vi "WaveGraph_Facade.vi"(0 "Data In":T5 caption="数据输入", 2 "Display State In":T3 caption="显示状态输入", 3 "Container State":T4 caption="容器状态") -> (6 "Data Out":T5 caption="数据输出", 7 "Display State Out":T3 caption="显示状态输出", 8 "Action":T2 caption="动作")   [LabVIEW 2012, in "WaveGraphX.xctl"]
uses:
  WaveGraphX.xctl
  WaveGrpah_Data.ctl
  <vilib>/_xctls/Container State.ctl
  WaveGraph_State.ctl
  <vilib>/Utility/miscctls.llb/LVPoint32TypeDef.ctl
  <vilib>/_xctls/Action.ctl
  <vilib>/_xctls/XControlSupport.lvlib
panel:
  out "峰值图例拖动State":bool
  out "统计图例拖动State":bool
  out "峰值图例":picture
  out "统计图例":picture
  out "图例拖动State":bool
  out "图例":picture
  out "队列中元素数量":i32
  in  "图例拖动坐标队列":refnum<queue>
  out "坐标 2":T1 caption="坐标"
  out "项标识符":string
  out "WaveForm Graph":dbl[](graph)
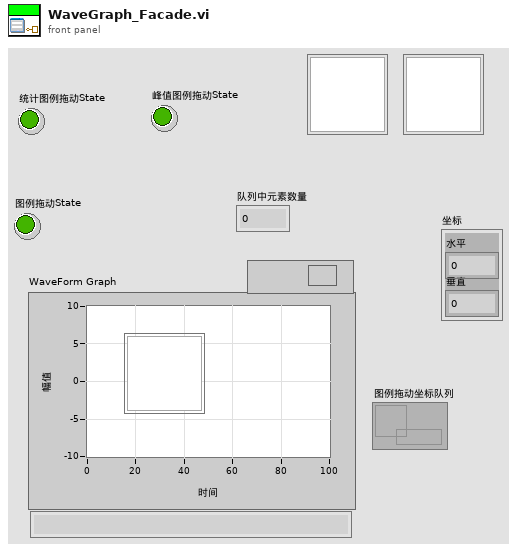
[diagram p1: front panel]
types:
  T1 = typedef "LVPoint32TypeDef.ctl" = cluster{"Horizontal":i32, "Vertical":i32}
  T2 = typedef "XControlSupport.lvlib/Action.ctl" = cluster{"Data Changed?":bool, "State Changed?":bool, "Action Name":string}
  T3 = typedef "WaveGraphX.xctl/WaveGraph_State.ctl" = cluster{"图例拖动State":bool, "统计图例拖动State":bool, "峰值图例拖动State":bool, "图例拖动坐标 队列":refnum<queue>, "统计图例拖动坐标 队列":refnum<queue>, "峰值图例拖动坐标 队列":refnum<queue>, "后台服务VI 引用":refnum<vi>, "控件引用簇 队列":refnum<queue>}
  T4 = typedef "XControlSupport.lvlib/Container State.ctl" = cluster{"Indicator?":bool, "Run Mode?":bool, " Refnum":refnum<vi>}
  T5 = typedef "WaveGraphX.xctl/WaveGrpah_Data.ctl" = dbl[]
  T6 = cluster{"图例拖动State":refnum<vi>, "统计图例拖动State":refnum<vi>, "峰值图例拖动State":refnum<vi>, "图例":refnum<vi>, "统计图例":refnum<vi>, "峰值图例":refnum<vi>}
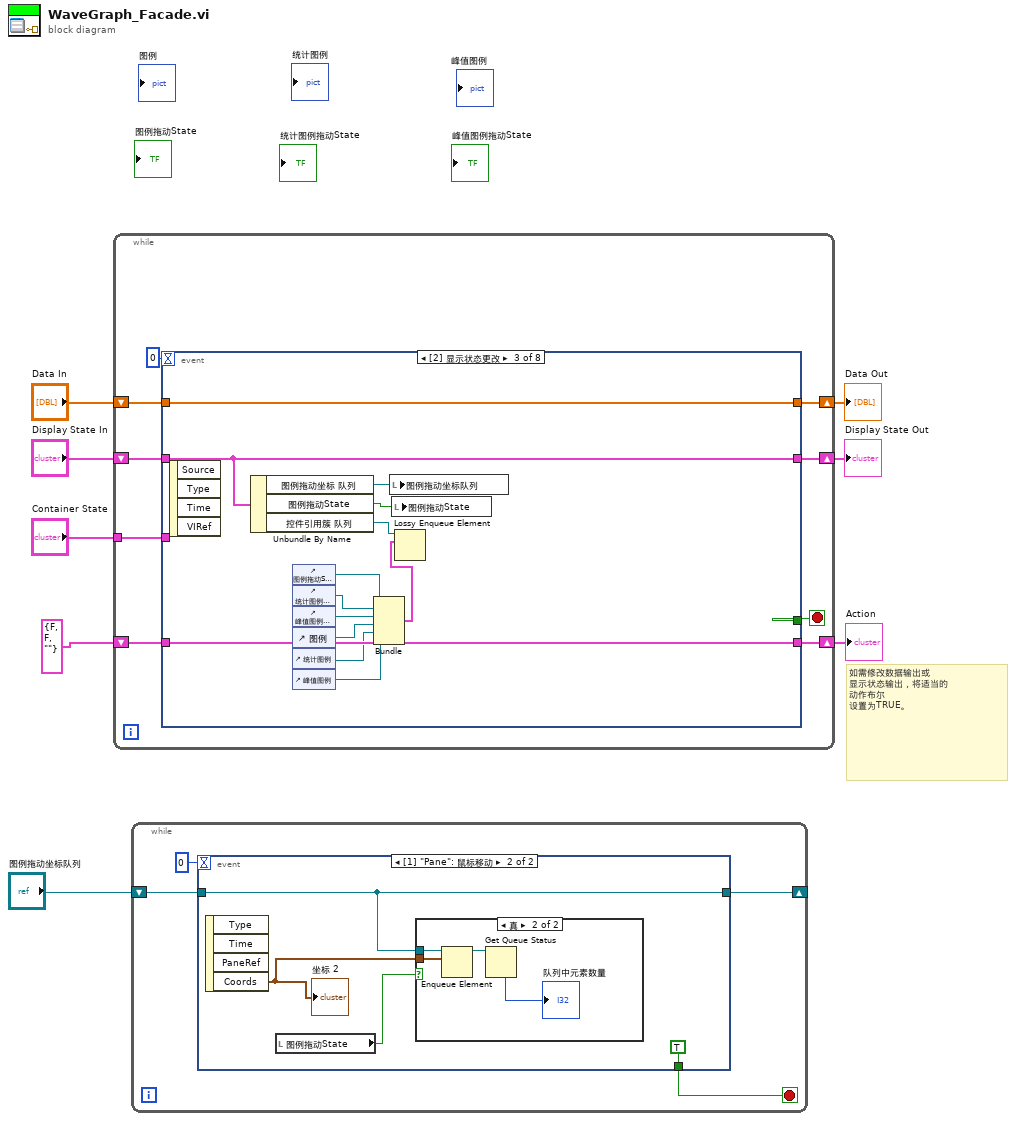
[diagram p0: block diagram]
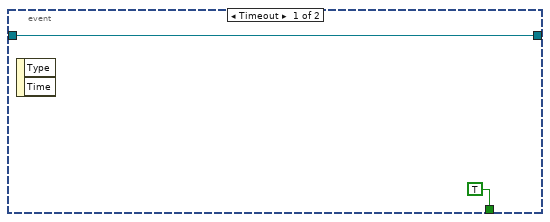
[diagram p2: hidden frame]
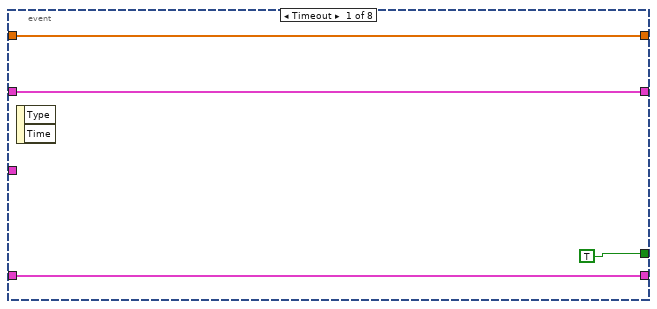
[diagram p4: hidden frame]
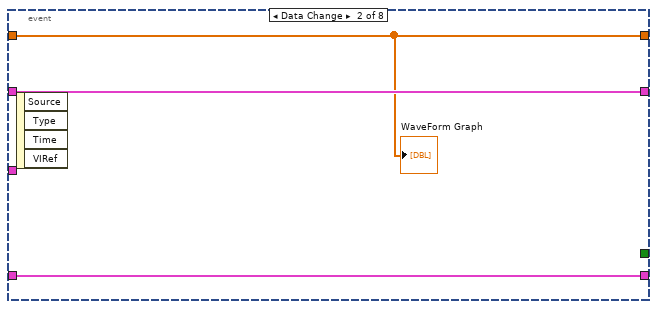
[diagram p5: hidden frame]
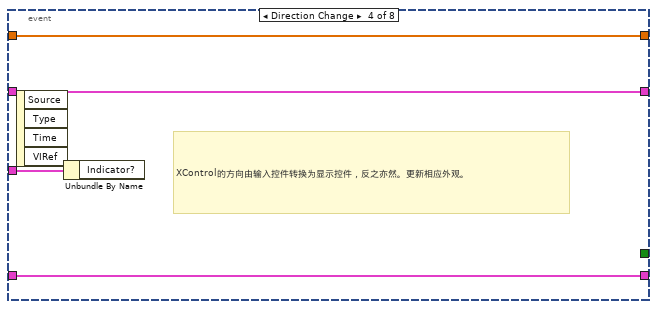
[diagram p6: hidden frame]
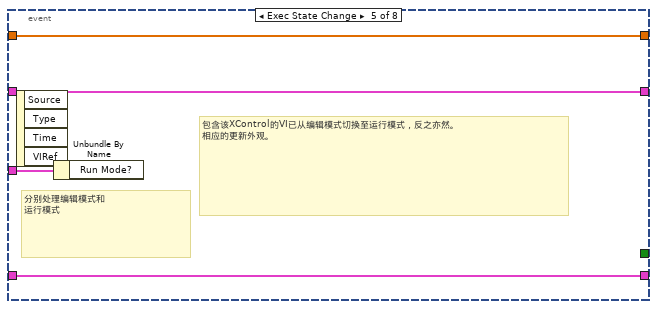
[diagram p7: hidden frame]
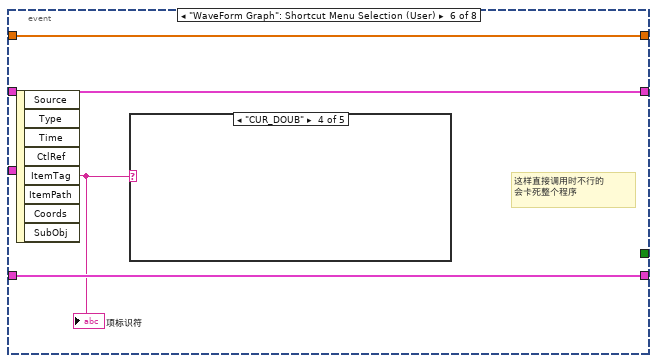
[diagram p8: hidden frame]
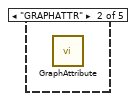
[diagram p10: hidden frame]
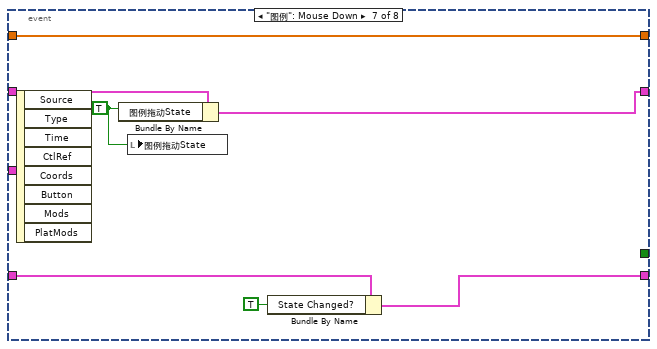
[diagram p13: hidden frame]
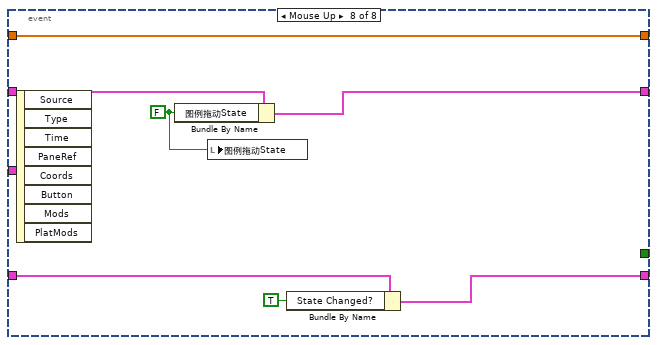
[diagram p14: hidden frame]
diagram:
  # "如需修改数据输出或\n显示状态输出，将适当的\n动作布尔\n设置为TRUE。"
  n1 = while {
    shift-right: [w16] -> w5
    shift-left: "Display State In" -> [w17]
    tunnel: "Container State" -> [w13]
    shift-right: [w11] -> w8
    shift-left: "Data In" -> [w12]
    shift-right: [w9] -> w3
    shift-left: T2 {"Data Changed?"=FALSE, "State Changed?"=FALSE, "Action Name"=""} ("Action") -> [w10]
    stop <- w15 stop-if-true
    n2 = event shown="[2] 显示状态更改" {
      selector: _ -> [_ _ _ _ _ _ _ _]
      dyn-events: _ -> [_ _ _ _ _ _ _ _]
      timeout: 0 -> [_ _ _ _ _ _ _ _]
      tunnel: w17 -> [w19 w24 w35 w40 w44 w49 w56 w62]
      tunnel: [w19 w24 w35 w40 w44 w49 w54 w61] -> w16
      tunnel: [TRUE _ _ _ _ _ _ _] -> w15
      tunnel: w13 -> [_ _ _ w41 w45 _ _ _]
      tunnel: w12 -> [w18 w22 w37 w39 w43 w48 w55 w63]
      tunnel: [w18 w22 w37 w39 w43 w48 w55 w63] -> w11
      tunnel: [w20 w23 w36 w38 w42 w47 w52 w59] -> w9
      tunnel: w10 -> [w20 w23 w36 w38 w42 w47 w53 w60]
      event Timeout {
        n3 = event-data() -> ()  [unwired: 1 in, 2 out]
      }
      event Data Change {
        n4 = event-data() -> ()  [unwired: 1 in, 4 out]
        "WaveForm Graph" <- w22
      }
      event Display State Change {
        n5 = event-data() -> ()  [unwired: 1 in, 4 out]
        n6 = Unbundle By Name(w35) -> ("图例拖动坐标 队列"=w34:refnum<queue>, "图例拖动State"=w33:bool, "控件引用簇 队列"=w32:refnum<queue>)
        n7 = control-ref of="图例拖动State"() -> (w26:refnum<vi>)
        n8 = control-ref of="统计图例拖动State"() -> (w27:refnum<vi>)
        n9 = control-ref of="峰值图例拖动State"() -> (w28:refnum<vi>)
        n10 = control-ref of="图例"() -> (w29:refnum<vi>)
        n11 = control-ref of="统计图例"() -> (w30:refnum<vi>)
        n12 = control-ref of="峰值图例"() -> (w31:refnum<vi>)
        n13 = Bundle("图例拖动State"=w26, "统计图例拖动State"=w27, "峰值图例拖动State"=w28, "图例"=w29, "统计图例"=w30, "峰值图例"=w31) -> (w25:T6)  [unwired: 1 in]
        n14 = local write "图例拖动坐标队列"(w34) -> ()
        n15 = local write "图例拖动State"(w33) -> ()
        n16 = Lossy Enqueue Element(queue=w32, element=w25) -> ()  [unwired: 1 in, 4 out]
      }
      event Direction Change {
        # "XControl的方向由输入控件转换为显示控件，反之亦然。更新相应外观。"
        n17 = event-data() -> ()  [unwired: 1 in, 4 out]
        n18 = Unbundle By Name(w41) -> ()  [unwired: 1 out]
      }
      event Exec State Change {
        # "包含该XControl的VI已从编辑模式切换至运行模式，反之亦然。\n相应的更新外观。"
        # "分别处理编辑模式和\n运行模式"
        n19 = event-data() -> ()  [unwired: 1 in, 4 out]
        n20 = Unbundle By Name(w45) -> ()  [unwired: 1 out]
      }
      event "WaveForm Graph": Shortcut Menu Selection (User) {
        # "这样直接调用时不行的\n会卡死整个程序"
        n21 = event-data() -> ("ItemTag"=w46:string)  [unwired: 1 in, 7 out]
        "项标识符" <- w46
        n22 = case shown="\"CUR_DOUB\"" w46 {
          frame " ", Default {
          }
          frame "GRAPHATTR" {
            n23 = call "GraphAttribute.vi"() -> ()  [unwired: 12 in]
          }
          frame "CUR_SING" {
          }
          frame "CUR_DOUB" {
          }
          frame "CUR_PEAK" {
          }
        }
      }
      event "图例": Mouse Down {
        w50 = TRUE ("图例拖动State")
        n24 = event-data() -> ()  [unwired: 1 in, 8 out]
        n25 = Bundle By Name(cluster=w56, "图例拖动State"=w50) -> (w54:T3)
        n26 = local write "图例拖动State"(w50) -> ()
        n27 = Bundle By Name(cluster=w53, "State Changed?"=TRUE) -> (w52:T2)
      }
      event Mouse Up {
        w57 = FALSE ("图例拖动State")
        n28 = event-data() -> ()  [unwired: 1 in, 8 out]
        n29 = Bundle By Name(cluster=w62, "图例拖动State"=w57) -> (w61:T3)
        n30 = local write "图例拖动State"(w57) -> ()
        n31 = Bundle By Name(cluster=w60, "State Changed?"=TRUE ("Data Changed?")) -> (w59:T2)
      }
    }
  }
  "Display State Out" <- w5
  "Data Out" <- w8
  "Action" <- w3
  n32 = while {
    shift-right: [w64] -> _
    shift-left: "图例拖动坐标队列" -> [w65]
    stop <- w66 stop-if-true
    n33 = event shown="[1] \"Pane\": 鼠标移动" {
      selector: _ -> [_ _]
      dyn-events: _ -> [_ _]
      timeout: 0 -> [_ _]
      tunnel: [TRUE TRUE] -> w66
      tunnel: w65 -> [w68 w72]
      tunnel: [w68 w72] -> w64
      event Timeout {
        n34 = event-data() -> ()  [unwired: 1 in, 2 out]
      }
      event Mouse Move {
        n35 = event-data() -> ("Coords"=w71:T1)  [unwired: 1 in, 3 out]
        "坐标 2" <- w71
        n36 = local read "图例拖动State"() -> (w70:bool)
        n37 = case shown="真" w70 {
          tunnel: w72 -> [_ w77]
          tunnel: w71 -> [_ w76]
          frame False {
          }
          frame True {
            n38 = Enqueue Element(queue=w77, element=w76) -> (queue out=w75:refnum<queue>)  [unwired: 2 in, 2 out]
            n39 = Get Queue Status(queue=w75) -> (# elements in queue=→"队列中元素数量":i32)  [unwired: 2 in, 7 out]
          }
        }
      }
    }
  }
